vi "Add_Part_of_Track(After_11)_Problem-1.vi"(4 "[IN] Index in subtrack":i32, 5 "[IN] Minimal Sub\ntrack Length":i32, 6 "[IN] Subtrack":T2, 7 "[IN] Indexes for Jumps":i32[](array[numeric]), 8 "error IN":errorcluster, 9 "[IN] Count of variants":i32, 10 "[IN] Subtracks":T1(array[cluster]), 11 "[IN] Still connected\ntracks in group":T3) -> (0 "error OUT":errorcluster, 1 "[OUT] Count of variants":i32, 2 "[OUT] Subtracks":T1(array[cluster]))   [LabVIEW 2013]
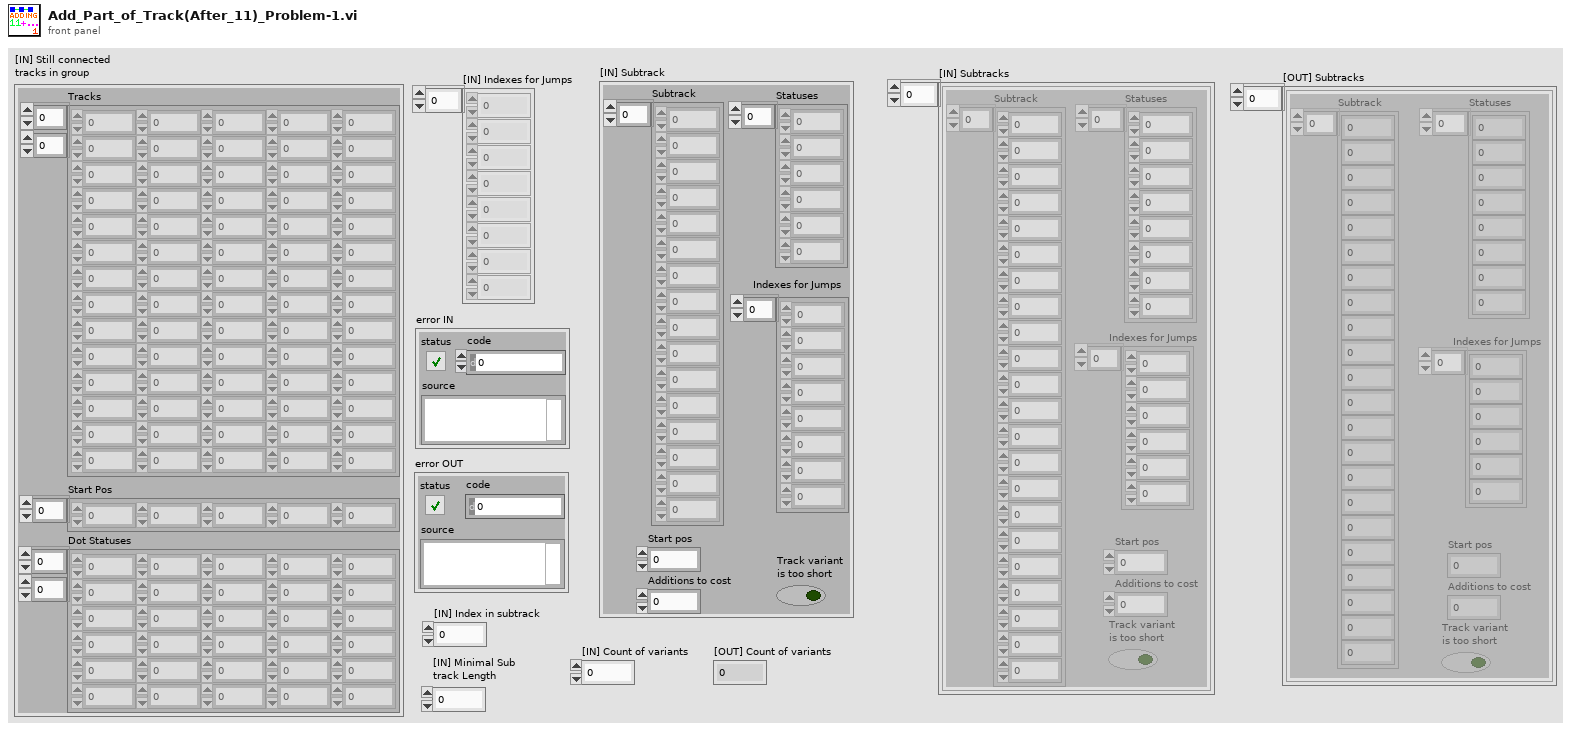
[diagram p1: front panel]
types:
  T1 = cluster{"Subtrack":dbl[], "Statuses":i16[], "Start pos":i32, "Additions to cost":i32, "Track variant \nis too short":bool, "Indexes for Jumps":i32[]}[]
  T2 = cluster{"Subtrack":dbl[], "Statuses":i16[], "Start pos":i32, "Additions to cost":i32, "Track variant \nis too short":bool, "Indexes for Jumps":i32[]}
  T3 = cluster{"Tracks":dbl[][], "Start Pos":i32[], "Dot Statuses":i16[][]}
  T4 = cluster{"Subtrack":dbl[], "Statuses":i16[], "Start pos":i32, "Additions to cost":i8, "Track variant \nis too short":bool, "Indexes for Jumps":i32[]}
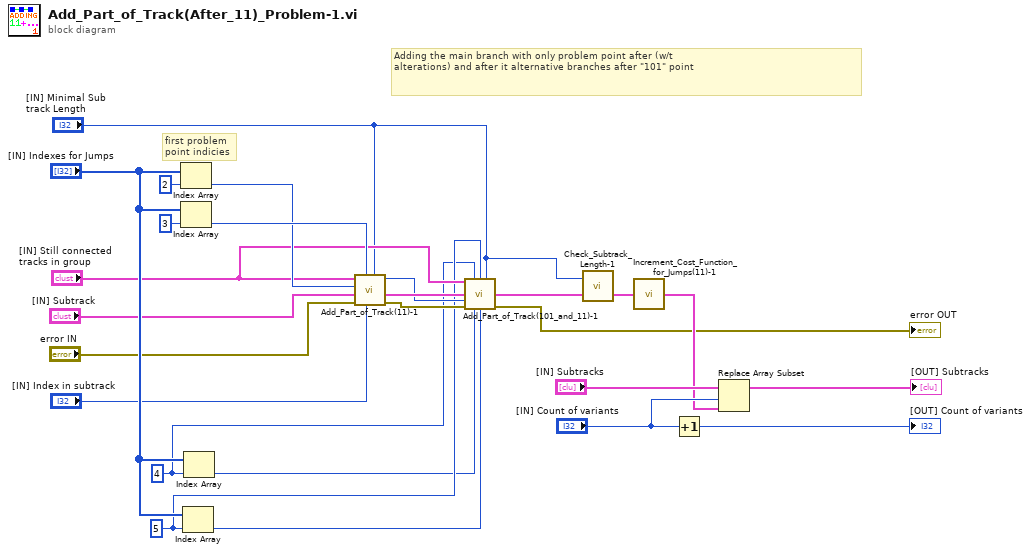
[diagram p0: block diagram]
diagram:
  w7 = 5 ("index")
  w6 = 4 ("index")
  # "first problem \npoint indicies"
  # "Adding the main branch with only problem point after (w/t \nalterations) and after it alternative branches after \"101\" point"
  n1 = Index Array(array="[IN] Indexes for Jumps", index=2) -> (element=w15:i32)
  n2 = Index Array(array="[IN] Indexes for Jumps", index=3) -> (element=w16:i32)
  n3 = Index Array(array="[IN] Indexes for Jumps", index=w7) -> (element=w4:i32)
  n4 = Index Array(array="[IN] Indexes for Jumps", index=w6) -> (element=w3:i32)
  n5 = call "Add_Part_of_Track(11)-1.vi"("[IN] Minimal Sub\ntrack Length"="[IN] Minimal Sub\ntrack Length", "[IN] Index in subtrack"="[IN] Index in subtrack", "[IN] # of subtrack conta\nining problem point"=w16, "error IN"="error IN", "[IN] Subtrack"="[IN] Subtrack", "[IN] Index of problem\npoint inside subtrack"=w15, "[IN] Still connected\ntracks in group"="[IN] Still connected\ntracks in group") -> ("error OUT"=w8:errorcluster, "[OUT] Subtrack"=w10:T2, "[OUT] Last point in subtrack"=w9:i32)  [unwired: 2 in]
  n6 = call "Add_Part_of_Track(101_and_11)-1.vi"("[IN] Still connected\ntracks in group"="[IN] Still connected\ntracks in group", "[IN] i for Probl\nem  Point Index"=w6, "[IN] i for # of Track \nwith Problem Point"=w7, "[IN] Minimal Sub\ntrack Length"="[IN] Minimal Sub\ntrack Length", "[IN] Subtrack"=w10, "[IN] Index in subtrack"=w9, "error IN"=w8, "[IN] Index of problem\npoint inside subtrack"=w3, "[IN] # of subtrack conta\nining problem point"=w4) -> ("[OUT] Subtrack"=w2:T2, "error OUT"=→"error OUT":errorcluster)  [unwired: 4 in, 1 out]
  n7 = call "Check_Subtrack_Length-1.vi"("[IN] Subtrack"=w2, "[IN] Minimal Sub\ntrack Length"="[IN] Minimal Sub\ntrack Length") -> ("[OUT] Subtrack"=w18:T4)  [unwired: 1 in]
  n8 = call "Increment_Cost_Function_for_Jumps(11)-1.vi"("[IN] Subtrack"=w18) -> ("[OUT] Subtrack"=w17:T2)
  n9 = Increment(x="[IN] Count of variants") -> (x+1=→"[OUT] Count of variants":i32)
  n10 = Replace Array Subset(array="[IN] Subtracks", new element=w17, index="[IN] Count of variants") -> (→"[OUT] Subtracks":T1)
